vi "get #OfImages.vi"(8 "error in (no error)":errorcluster, 11 "Segment in":refnum<class "Test.lvclass">) -> (0 "error out":errorcluster, 2 "#OfImages":u32, 3 "Segment out":refnum<class "Test.lvclass">)   [LabVIEW 2013]
uses:
  Test.lvclass
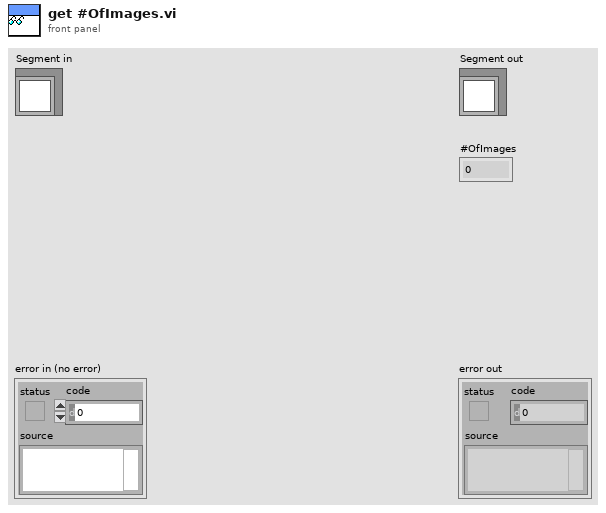
[diagram p1: front panel]
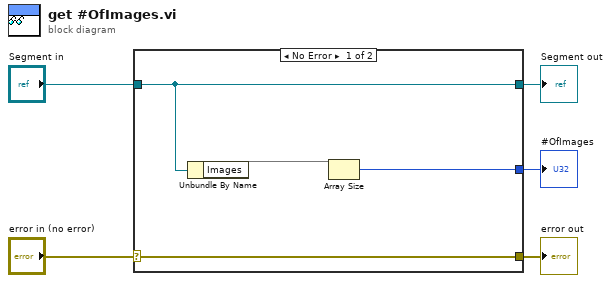
[diagram p0: block diagram]
diagram:
  n1 = case shown="No Error" "error in (no error)" {
    selector: "error in (no error)" -> [w9 w10]
    tunnel: [w9 w10] -> w4
    tunnel: [w8 w11] -> w2
    tunnel: "Segment in" -> [w8 w11]
    tunnel: [w6 _] -> w1
    frame No Error {
      n2 = Unbundle By Name(w8) -> ("Images"=w7)
      n3 = Array Size(array=w7) -> (size(s)=w6:i32)
    }
    frame Error {
    }
  }
  "error out" <- w4
  "Segment out" <- w2
  "#OfImages" <- w1
